vi "Determine Warnings.vi"(8 "Error In":errorcluster, 10 "Weather Data In":T1) -> (0 "Error Out":errorcluster, 2 "Weather Data Out":T1)   [LabVIEW 2020]
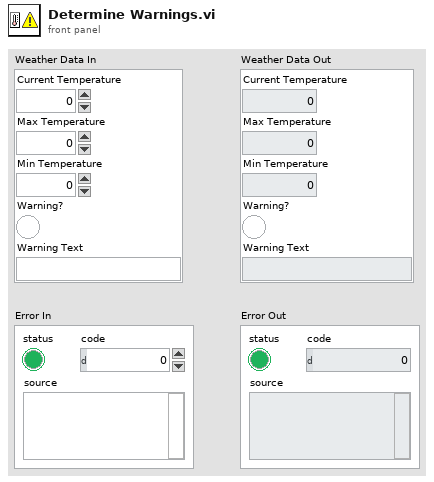
[diagram p1: front panel]
types:
  T1 = cluster{"Current Temperature":dbl, "Max Temperature":dbl, "Min Temperature":dbl, "Warning?":bool, "Warning Text":string}
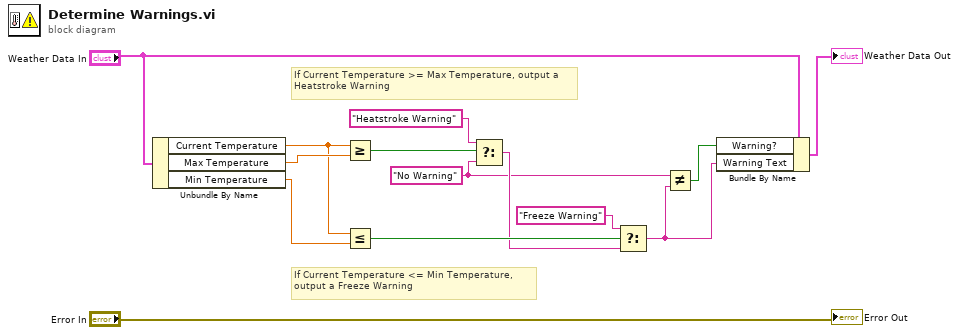
[diagram p0: block diagram]
diagram:
  w6 = "No Warning"
  # "If Current Temperature <= Min Temperature, output a Freeze Warning"
  # "If Current Temperature >= Max Temperature, output a Heatstroke Warning"
  n1 = Unbundle By Name("Weather Data In") -> ("Current Temperature"=w13:dbl, "Max Temperature"=w14:dbl, "Min Temperature"=w12:dbl)
  n2 = Greater Or Equal?(x=w13, y=w14) -> (x >= y?=w11:bool)
  n3 = Less Or Equal?(x=w13, y=w12) -> (x <= y?=w9:bool)
  n4 = Select(t="Heatstroke Warning", s=w11, f=w6) -> (s? t:f=w7:string)
  n5 = Select(t="Freeze Warning", s=w9, f=w7) -> (s? t:f=w4:string)
  n6 = Not Equal?(x=w6, y=w4) -> (x != y?=w5:bool)
  n7 = Bundle By Name(cluster="Weather Data In", "Warning?"=w5, "Warning Text"=w4) -> (→"Weather Data Out":T1)
  "Error Out" <- "Error In"
